vi "Get Module Type Info.vi"(11 "error in (no error)":errorcluster) -> (4 "ModuleTypes":string[](array[string]), 15 "error out":errorcluster)   [LabVIEW 2020, in "DQMH_API.lvclass"]
uses:
  <resource>/Framework/Providers/Open_GDS/UML/DQMH_API_class/DQMH_API.lvclass
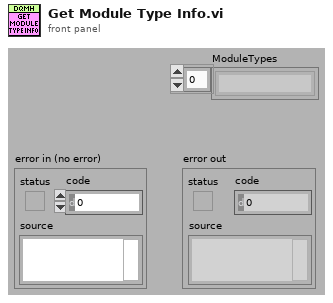
[diagram p1: front panel]
types:
  T1 = typedef "DQMH_API.lvclass/ObjectAttributes.ctl" = cluster{"Get Module Type Info":refnum<vi>, "Script New Module":refnum<vi>, "Script New Event":refnum<vi>, "Query Library for Module Info":refnum<vi>, "Parse Project for DQMH Modules":refnum<vi>, "Get All Events in Module":refnum<vi>}
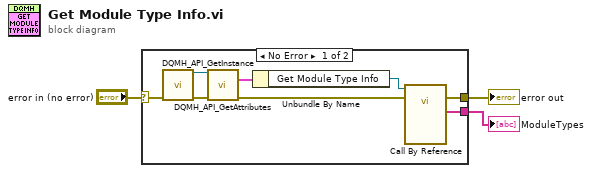
[diagram p0: block diagram]
diagram:
  n1 = case shown="No Error" "error in (no error)" {
    selector: "error in (no error)" -> [w9 w12]
    tunnel: [w5 w12] -> w2
    tunnel: [w4 _] -> w1
    frame No Error {
      n2 = call <resource>:"DQMH_API_GetInstance.vi"("error in (no error)"=w9) -> ("reference out"=w10:refnum<class "DQMH_API.lvclass">, "error out"=w8:errorcluster)  [unwired: 10 in, 3 out]
      n3 = call <resource>:"DQMH_API_GetAttributes.vi"("reference in"=w10, "error in (no error)"=w8) -> ("Data"=w11:T1, "error out"=w6:errorcluster)  [unwired: 10 in, 2 out]
      n4 = Unbundle By Name(w11) -> ("Get Module Type Info"=w7:refnum<vi>)
      n5 = call-by-ref "?"(reference=w7, error in=w6) -> (error out=w5:errorcluster, "ModuleTypes"=w4:string[])  [unwired: 11 in, 1 out]
    }
    frame Error {
    }
  }
  "error out" <- w2
  "ModuleTypes" <- w1
